vi "Histograma.vi"() -> ()   [LabVIEW 2020]
uses:
  <vilib>/Instr/_visa.llb/VISA Configure Serial Port (Instr).vi
  <vilib>/Analysis/NI_AALBase.lvlib
panel:
  in  "stop":bool
  out "Histogram Graph":T1(graph)
  out "read buffer":string
  out "number":i32
  in  "VISA resource name":refnum<visa-resource-name>
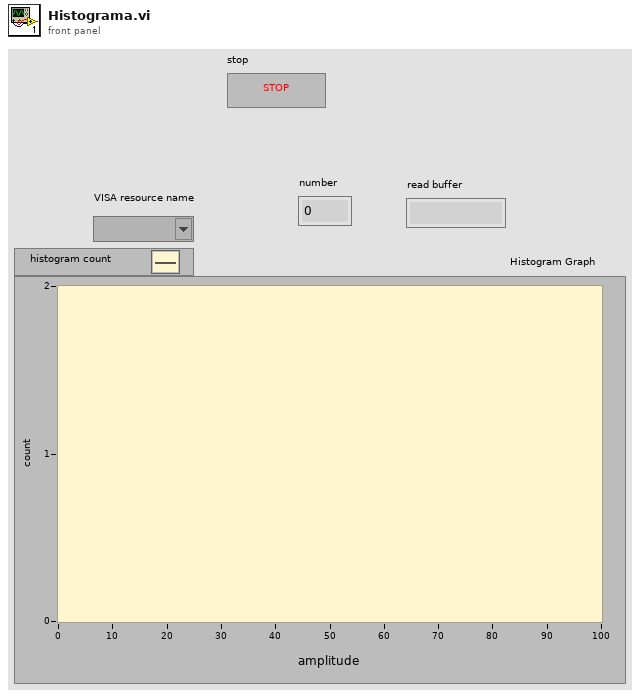
[diagram p1: front panel]
types:
  T1 = cluster{"X Values":dbl[], "Histogram: h(x)":i32[]}
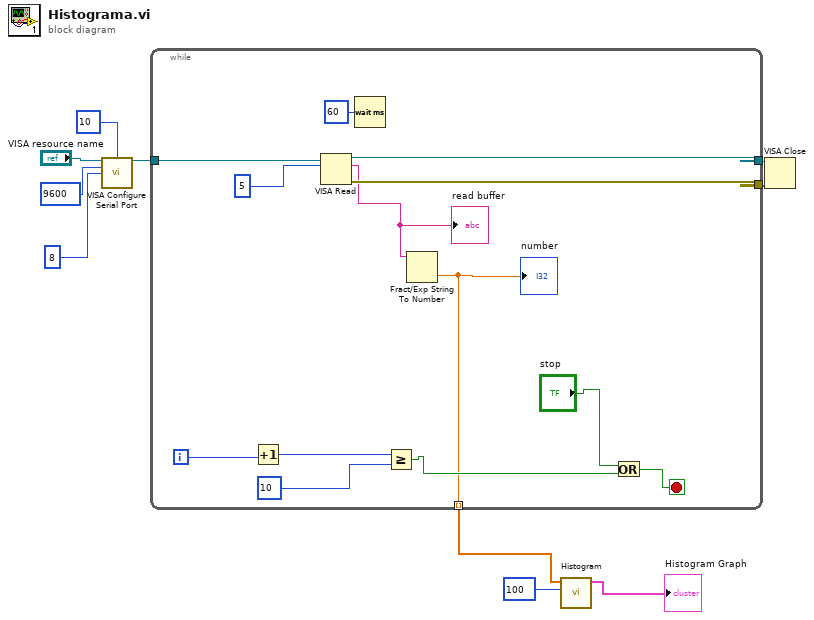
[diagram p0: block diagram]
diagram:
  n1 = call-poly "VISA Configure Serial Port"("VISA resource name"="VISA resource name", "termination char\n(0xA = '\\n' = LF)"=u8 10 ("termination char\n(0xA = '\\n' = LF)"), "baud rate (9600)"=u32 9600, "data bits (8)"=u16 8) -> ("VISA resource name out"=w10:refnum<visa-resource-name>)  [unwired: 10 in, 1 out]
  n2 = while {
    tunnel: w10 -> [w15]
    tunnel: [w23] -> w5
    tunnel: [w21] -> w6
    tunnel: [w11] -> w3 mode=indexing
    i -> [w13]
    stop <- w18 stop-if-true
    n3 = Increment(x=w13) -> (x+1=w12:i32)
    n4 = VISA Read(VISA resource name=w15, byte count=u32 5) -> (VISA resource name out=w23:refnum<visa-resource-name>, read buffer=w20:string, error out=w21:errorcluster)  [unwired: 1 in, 1 out]
    "read buffer" <- w20
    n5 = Wait (ms)(milliseconds to wait=u32 60) -> ()  [unwired: 1 out]
    n6 = Greater Or Equal?(x=w12, y=10) -> (x >= y?=w16:bool)
    n7 = Fract/Exp String To Number(string=w20) -> (number=w11:dbl)  [unwired: 3 in, 1 out]
    "number" <- w11
    n8 = Or(x="stop", y=w16) -> (x .or. y?=w18:bool)
  }
  n9 = call <vilib>:"Histogram.vi"("intervals"=100, "X"=w3) -> ("Histogram Graph"=→"Histogram Graph":T1)  [unwired: 6 in, 3 out]
  n10 = VISA Close(VISA resource name=w5, error in (no error)=w6) -> ()  [unwired: 1 out]
